vi "Index Array Elements - error cluster.vi"(4 "indices (none)":i32[](array[numeric])=[3, -1, 4], 7 "1D Array":errorcluster[](array[cluster])) -> (0 "output array":errorcluster[](array[cluster]))   [LabVIEW 2020]
doc: "Returns the elements of a 1-dimension array at indices. This is a list-based version of the built-in \"Index Array\"."
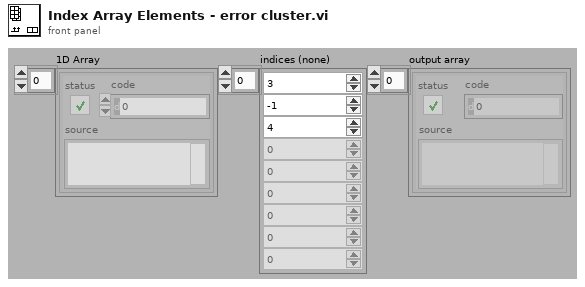
[diagram p1: front panel]
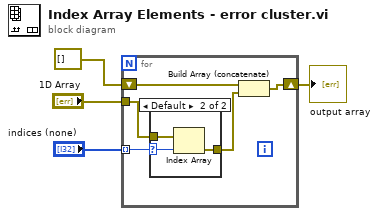
[diagram p0: block diagram]
diagram:
  n1 = for {
    shift-right: [w6] -> w3
    shift-left: errorcluster[] [] ("indices (none)") -> [w8]
    tunnel: "indices (none)" -> [w5] mode=indexing
    tunnel: "1D Array" -> [w9]
    n2 = case shown="Default" w5 {
      selector: w5 -> [_ w10]
      tunnel: w9 -> [_ w12]
      tunnel: [_ w11] -> w7
      frame -1 {
      }
      frame Default {
        n3 = Index Array(array=w12, index=w10) -> (element=w11:errorcluster)
      }
    }
    n4 = Build Array (concatenate)(w8, w7) -> (w6:errorcluster[])
  }
  "output array" <- w3
